vi "DOTNET-error.vi"   [LabVIEW 2013, in "MaterialCharacterization.lvlib" / "MC-SM1000.lvclass"]
uses:
  MC-SM1000.lvclass
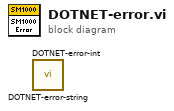
[diagram p0: block diagram]
diagram:
  n1 = call "DOTNET-error-string.vi"() -> ()  [unwired: 11 in, 1 out]
  n2 = call "DOTNET-error-int.vi"() -> ()  [unwired: 11 in, 1 out]
